vi "RGB.vi"() -> ()   [LabVIEW 2016]
panel:
  out "Color":u32(colorbox)
  in  "B":u8(slide) scale=0.0..255.0
  in  "G":u8(slide) scale=0.0..255.0
  in  "R":u8(slide) scale=0.0..255.0
  # "ne"
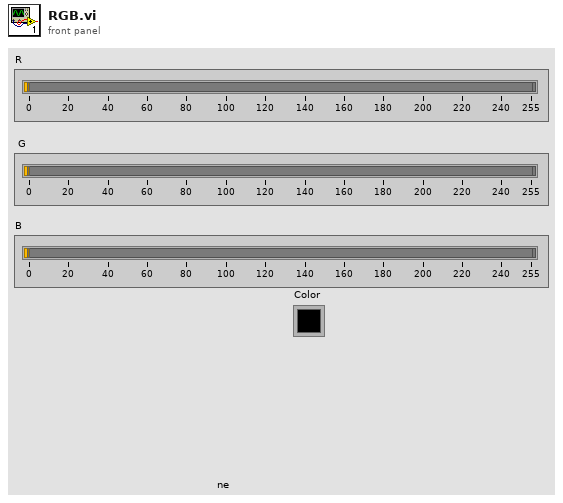
[diagram p1: front panel]
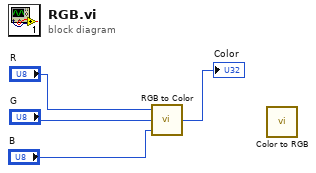
[diagram p0: block diagram]
diagram:
  n1 = call <vilib>:"RGB to Color.vi"("B"="B", "G"="G", "R"="R") -> ("Color"=→"Color":u32)
  n2 = call <vilib>:"Color to RGB.vi"() -> ()  [unwired: 1 in, 4 out]
